vi "LMB_WallFollow_SetHeading.vi"(8 "Follow Right?":bool=TRUE, 11 "Distance":i32) -> (3 "heading":i32)   [LabVIEW 2012]
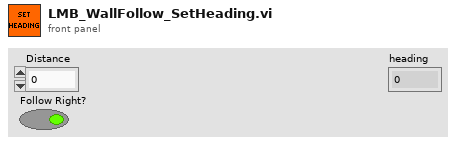
[diagram p1: front panel]
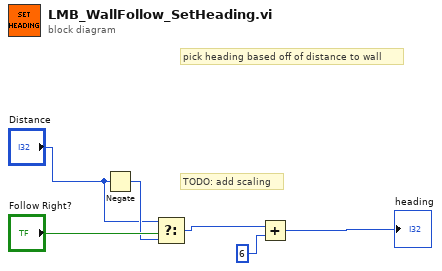
[diagram p0: block diagram]
diagram:
  # "pick heading based off of distance to wall"
  # "TODO: add scaling"
  n1 = Negate(x="Distance") -> (-x=w5:i32)
  n2 = Select(t="Distance", s="Follow Right?", f=w5) -> (s? t:f=w3:i32)
  n3 = Add(x=w3, y=6) -> (x+y=→"heading":i32)
